vi "Send Message Back To Self.vi"(8 "error in (no error)":errorcluster, 10 "Message In":refnum<class "Message.lvclass">, 11 "System Actor in":refnum<class "System Actor.lvclass">) -> (0 "error out":errorcluster, 3 "System Actor out":refnum<class "System Actor.lvclass">)   [LabVIEW 2024, in "System Actor.lvclass"]
uses:
  System Actor.lvclass
  Message/Message.lvclass
  System Actor.lvclass/System Actor.ctl
  Public Data/Call Messenger.vi
  Public Data/Read Self Messenger Location.vi
  Messenger/Messenger/Messenger.lvclass
  Messenger/Mail Strategy/Mail Strategy.lvclass
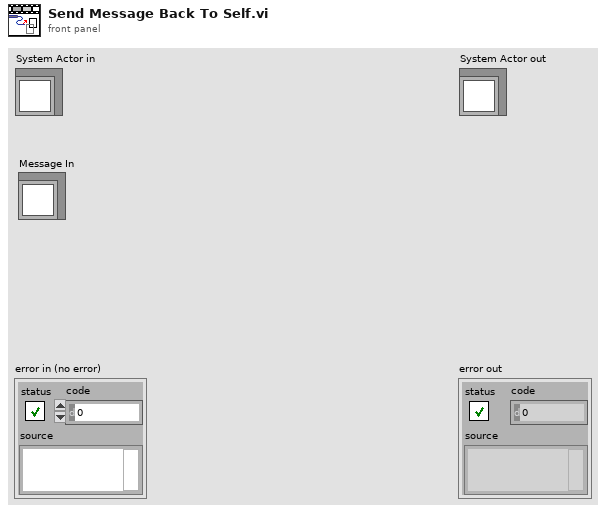
[diagram p1: front panel]
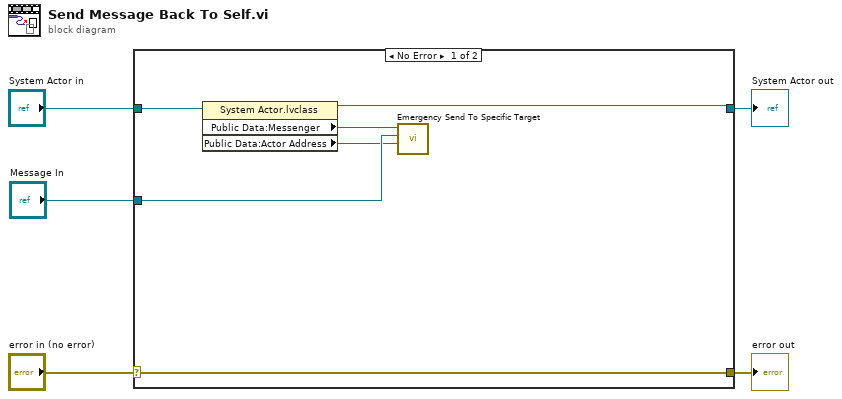
[diagram p0: block diagram]
diagram:
  n1 = case shown="No Error" "error in (no error)" {
    selector: "error in (no error)" -> [w11 w13]
    tunnel: [w11 w13] -> w4
    tunnel: [w9 w12] -> w2
    tunnel: "System Actor in" -> [w10 w12]
    tunnel: "Message In" -> [w7 _]
    frame No Error {
      n2 = property class="System Actor.lvclass"(reference=w10) -> (reference out=w9:refnum<class "System Actor.lvclass">, "Public Data:Messenger"=w8:refnum<class "Messenger.lvclass">, "Public Data:Actor Address"=w6:refnum<class "Mail Strategy.lvclass">)  [unwired: 1 in, 1 out]
      n3 = call-dynamic "Emergency Send To Specific Target.vi"("Mail Strategy In"=w6, "Message In"=w7, "Messenger in"=w8) -> ()  [unwired: 7 in, 2 out]
    }
    frame Error {
    }
  }
  "error out" <- w4
  "System Actor out" <- w2
